vi "cRIO_4DoF_Encoders_counts2rad(subVI).vi"() -> (1 "Theta3":dbl, 2 "Theta2":dbl, 3 "Theta1":dbl, 7 "Theta6":dbl)   [LabVIEW 2019]
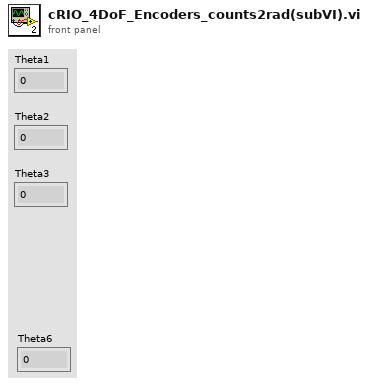
[diagram p1: front panel]
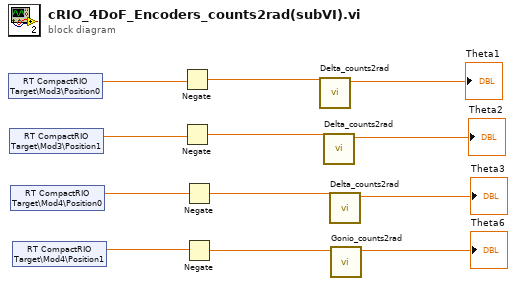
[diagram p0: block diagram]
diagram:
  n1 = shared-variable "RT CompactRIO Target\\Mod3\\Position0"() -> (w8:dbl)  [unwired: 1 in, 1 out]
  n2 = shared-variable "RT CompactRIO Target\\Mod3\\Position1"() -> (w6:dbl)  [unwired: 1 in, 1 out]
  n3 = shared-variable "RT CompactRIO Target\\Mod4\\Position0"() -> (w4:dbl)  [unwired: 1 in, 1 out]
  n4 = shared-variable "RT CompactRIO Target\\Mod4\\Position1"() -> (w2:dbl)  [unwired: 1 in, 1 out]
  n5 = Negate(x=w8) -> (-x=w7:dbl)
  n6 = Negate(x=w6) -> (-x=w5:dbl)
  n7 = Negate(x=w4) -> (-x=w3:dbl)
  n8 = Negate(x=w2) -> (-x=w1:dbl)
  n9 = call "Delta_counts2rad.vi"("Numeric in"=w7) -> ("Numeric"=→"Theta1":dbl)  [unwired: 10 in]
  n10 = call "Delta_counts2rad.vi"("Numeric in"=w5) -> ("Numeric"=→"Theta2":dbl)  [unwired: 10 in]
  n11 = call "Delta_counts2rad.vi"("Numeric in"=w3) -> ("Numeric"=→"Theta3":dbl)  [unwired: 10 in]
  n12 = call "Gonio_counts2rad.vi"("Numeric in"=w1) -> ("Numeric"=→"Theta6":dbl)  [unwired: 10 in]
